vi "坐标平移1D.vi"(8 "Error In":errorcluster caption="错误输入", 9 "dy":dbl, 10 "dx":dbl, 11 "输入点":T1[](array[typedef])) -> (0 "Error Out":errorcluster caption="错误输出", 3 "输出点":T1[](array[typedef]))   [LabVIEW 2012, in "几何工具.lvlib"]
uses:
  <vilib>/Utility/miscctls.llb/LVPointDoubleTypeDef.ctl
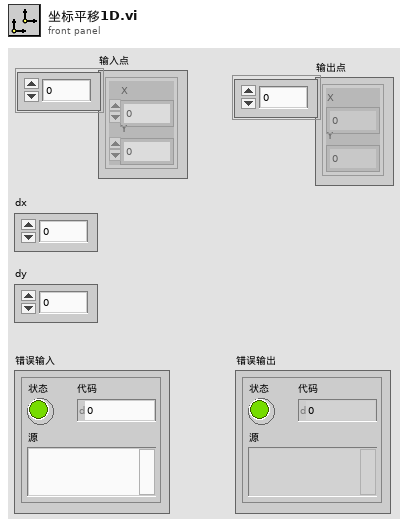
[diagram p1: front panel]
types:
  T1 = typedef "LVPointDoubleTypeDef.ctl" = cluster{"X":dbl, "Y":dbl}
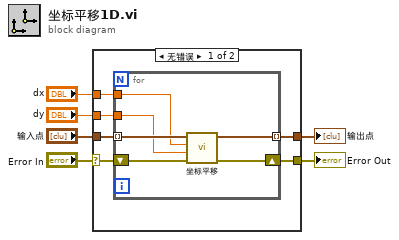
[diagram p0: block diagram]
diagram:
  n1 = case shown="无错误" "Error In" {
    selector: "Error In" -> [w8 w20]
    tunnel: [w7 w20] -> w5
    tunnel: "dx" -> [w10 _]
    tunnel: "dy" -> [w9 _]
    tunnel: "输入点" -> [w12 w19]
    tunnel: [w11 w19] -> w1
    frame No Error {
      n2 = for {
        tunnel: w12 -> [w18] mode=indexing
        tunnel: [w17] -> w11 mode=indexing
        tunnel: w10 -> [w16]
        tunnel: w9 -> [w15]
        shift-right: [w13] -> w7
        shift-left: w8 -> [w14]
        n3 = call-poly "坐标平移.vi"("Error In"=w14, "dy"=w15, "dx"=w16, "输入点"=w18) -> ("Error Out"=w13:errorcluster, "输出点"=w17:T1)  [unwired: 6 in]
      }
    }
    frame Error {
    }
  }
  "Error Out" <- w5
  "输出点" <- w1
